vi "apply_settings.vi"(0 "Handle":i32, 1 "PreAmp Gain Control":string(combo), 3 "Trigger mode":string, 5 "ExposureTime":dbl=0.1, 7 "ElectronicShutteringMode":string(combo), 9 "AOI Height":i64, 11 "AOI Width":i64, 12 "Centre AOI":bool) -> (4 "AOIStride":i64, 6 "ImageSizeBytes":i64, 10 "Pixel Encoding":string, 14 "PixelData":u16[](array[numeric]), 15 "ByteData":u8[](array[numeric]))   [LabVIEW 2019]
panel:
  in  "Apply Settings":bool
  out "Ready":bool
  in  "Run":bool
  in  "error":errorcluster
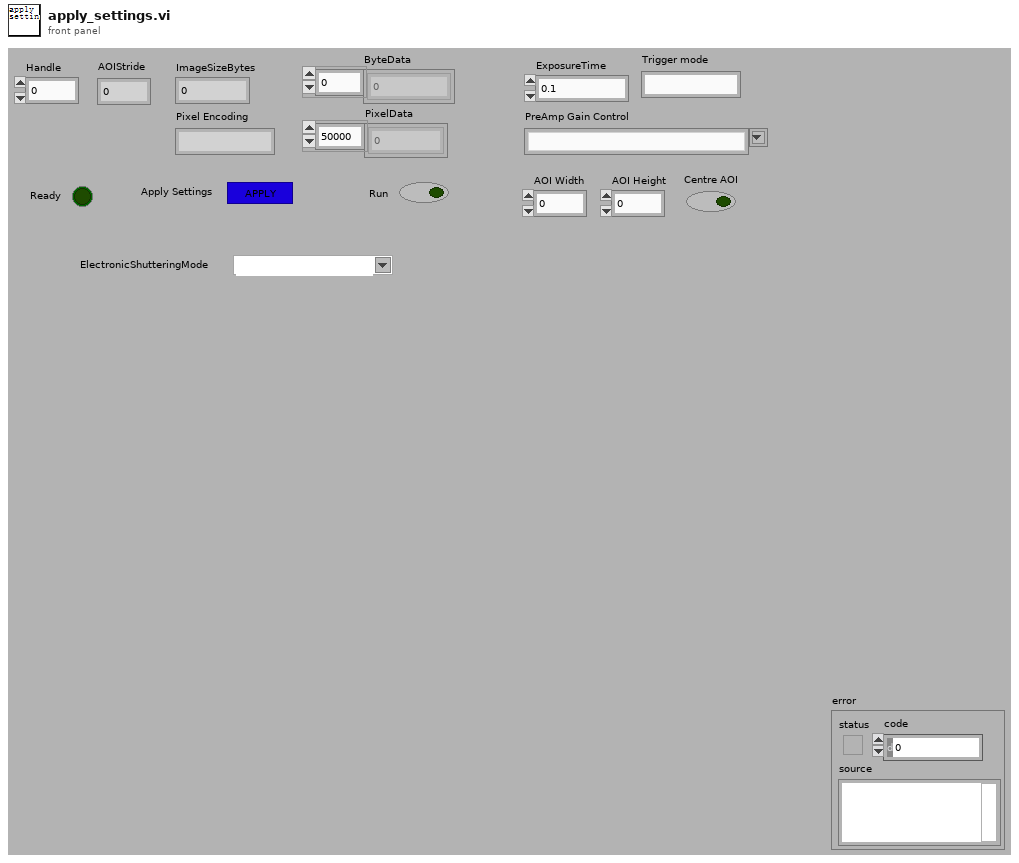
[diagram p1: front panel]
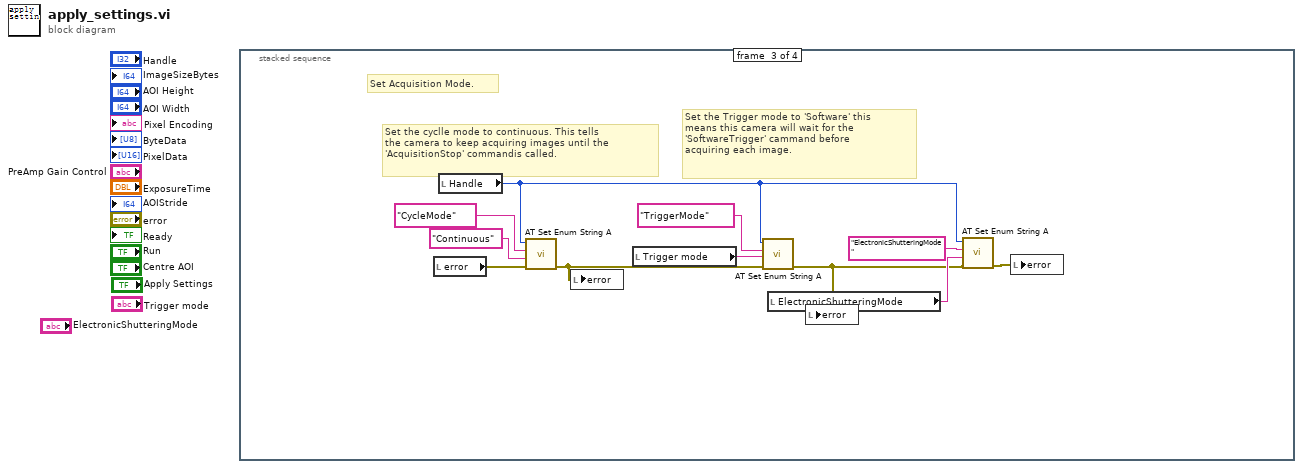
[diagram p0: block diagram]
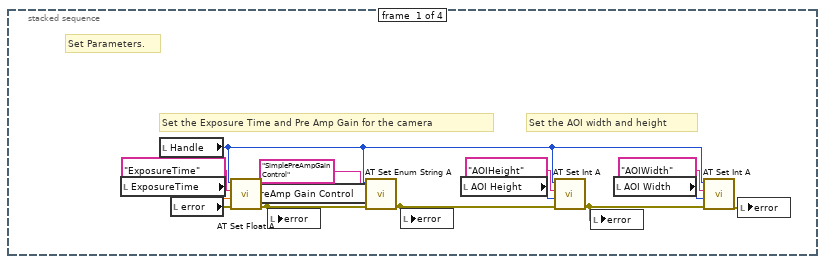
[diagram p2: hidden frame]
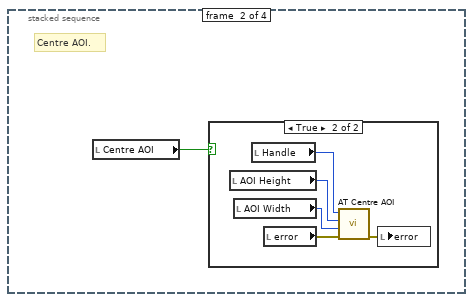
[diagram p3: hidden frame]
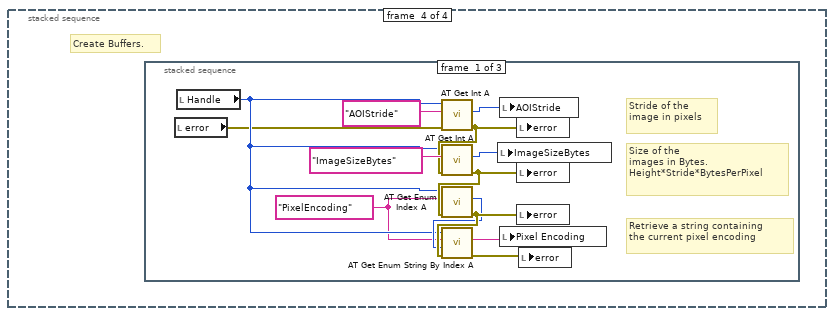
[diagram p5: hidden frame]
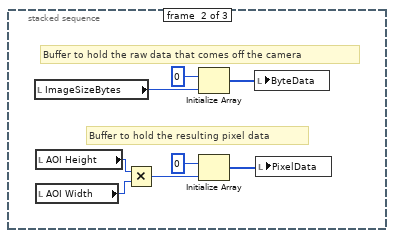
[diagram p6: hidden frame]
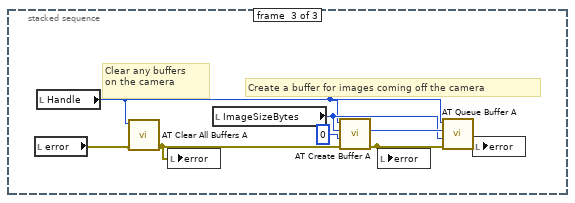
[diagram p7: hidden frame]
diagram:
  n1 = stacked-sequence {
    frame #0 {
      # "Set the AOI width and height"
      # "Set the Exposure Time and Pre Amp Gain for the camera"
      # "Set Parameters."
      n2 = local read "ExposureTime"() -> (w14:dbl)
      n3 = local read "Handle"() -> (w2:i32)
      n4 = local read "error"() -> (w10:errorcluster)
      n5 = call <userlib>:"AT Set Float A.vi"("error in (no error)"=w10, "Value"=w14, "Feature"="ExposureTime" ("ExposureTime"), "Hndl"=w2) -> ("error out"=w12:errorcluster)  [unwired: 6 in, 1 out]
      n6 = local read "PreAmp Gain Control"() -> (w13:string)
      n7 = local write "error"(w12) -> ()
      n8 = call <userlib>:"AT Set Enum String A.vi"("error in (no error)"=w12, "String"=w13, "Feature"="SimplePreAmpGainControl" ("Enum feature"), "Handle"=w2) -> ("error out"=w9:errorcluster)  [unwired: 6 in, 1 out]
      n9 = local write "error"(w9) -> ()
      n10 = local read "AOI Height"() -> (w6:i64)
      n11 = call <userlib>:"AT Set Int A.vi"("error in (no error)"=w9, "Value"=w6, "Feature"="AOIHeight" ("Integer feature"), "Handle"=w2) -> ("error out"=w7:errorcluster)  [unwired: 6 in, 1 out]
      n12 = local write "error"(w7) -> ()
      n13 = local read "AOI Width"() -> (w5:i64)
      n14 = call <userlib>:"AT Set Int A.vi"("error in (no error)"=w7, "Value"=w5, "Feature"="AOIWidth" ("Integer feature 2"), "Handle"=w2) -> ("error out"=w8:errorcluster)  [unwired: 6 in, 1 out]
      n15 = local write "error"(w8) -> ()
    }
    frame #1 {
      # "Centre AOI."
      n16 = local read "Centre AOI"() -> (w15:bool)
      n17 = case shown="True" w15 {
        frame False {
        }
        frame True {
          n18 = local read "AOI Height"() -> (w17:i64)
          n19 = local read "AOI Width"() -> (w18:i64)
          n20 = local read "Handle"() -> (w16:i32)
          n21 = local read "error"() -> (w19:errorcluster)
          n22 = call <userlib>:"AT Centre AOI.vi"("error in (no error)"=w19, "AOI Width"=w18, "AOI Height"=w17, "Handle"=w16) -> ("error out"=w20:errorcluster)  [unwired: 7 in]
          n23 = local write "error"(w20) -> ()
        }
      }
    }
    frame #2 {
      # "Set the Trigger mode to 'Software' this \nmeans this camera will wait for the \n'SoftwareTrigger' cammand before \nacquiring each image."
      # "Set the cyclle mode to continuous. This tells \nthe camera to keep acquiring images until the \n'AcquisitionStop' commandis called."
      # "Set Acquisition Mode."
      n24 = local read "error"() -> (w30:errorcluster)
      n25 = local read "Handle"() -> (w21:i32)
      n26 = call <userlib>:"AT Set Enum String A.vi"("error in (no error)"=w30, "String"="Continuous", "Feature"="CycleMode" ("Enum feature"), "Handle"=w21) -> ("error out"=w29:errorcluster)  [unwired: 6 in, 1 out]
      n27 = local write "error"(w29) -> ()
      n28 = local read "Trigger mode"() -> (w26:string)
      n29 = call <userlib>:"AT Set Enum String A.vi"("error in (no error)"=w29, "String"=w26, "Feature"="TriggerMode" ("Enum feature"), "Handle"=w21) -> ("error out"=w22:errorcluster)  [unwired: 6 in, 1 out]
      n30 = local read "ElectronicShutteringMode"() -> (w24:string)
      n31 = local write "error"(w22) -> ()
      n32 = call <userlib>:"AT Set Enum String A.vi"("error in (no error)"=w22, "String"=w24, "Feature"="ElectronicShutteringMode" ("Enum feature"), "Handle"=w21) -> ("error out"=w23:errorcluster)  [unwired: 6 in, 1 out]
      n33 = local write "error"(w23) -> ()
    }
    frame #3 {
      # "Create Buffers."
      n34 = stacked-sequence {
        frame #0 {
          w32 = "PixelEncoding" ("Enum feature")
          # "Retrieve a string containing \nthe current pixel encoding"
          # "Stride of the\nimage in pixels"
          # "Size of the\nimages in Bytes.\nHeight*Stride*BytesPerPixel"
          n35 = local read "error"() -> (w33:errorcluster)
          n36 = local read "Handle"() -> (w34:i32)
          n37 = call <userlib>:"AT Get Int A.vi"("error in (no error)"=w33, "Feature"="AOIStride" ("Integer feature"), "Handle"=w34) -> ("error out"=w40:errorcluster, "Value"=w44:i64)  [unwired: 6 in, 1 out]
          n38 = call <userlib>:"AT Get Int A.vi"("error in (no error)"=w40, "Feature"="ImageSizeBytes" ("Integer feature"), "Handle"=w34) -> ("error out"=w39:errorcluster, "Value"=w43:i64)  [unwired: 6 in, 1 out]
          n39 = call <userlib>:"AT Get Enum Index A.vi"("error in (no error)"=w39, "Feature"=w32, "Handle"=w34) -> ("error out"=w38:errorcluster, "Value"=w37:i32)  [unwired: 6 in, 1 out]
          n40 = call <userlib>:"AT Get Enum String By Index A.vi"("error in (no error)"=w38, "Index"=w37, "Feature"=w32, "Handle"=w34) -> ("error out"=w35:errorcluster, "String"=w36:string)  [unwired: 5 in, 1 out]
          n41 = local write "ImageSizeBytes"(w43) -> ()
          n42 = local write "AOIStride"(w44) -> ()
          n43 = local write "Pixel Encoding"(w36) -> ()
          n44 = local write "error"(w40) -> ()
          n45 = local write "error"(w39) -> ()
          n46 = local write "error"(w38) -> ()
          n47 = local write "error"(w35) -> ()
        }
        frame #1 {
          # "Buffer to hold the resulting pixel data"
          # "Buffer to hold the raw data that comes off the camera"
          n48 = local read "ImageSizeBytes"() -> (w46:i64)
          n49 = local read "AOI Height"() -> (w50:i64)
          n50 = local read "AOI Width"() -> (w51:i64)
          n51 = Multiply(x=w50, y=w51) -> (x*y=w45:i64)
          n52 = Initialize Array(u8 0, w46) -> (w48:u8[])
          n53 = Initialize Array(i64 0, w45) -> (w49:i64[])
          n54 = local write "ByteData"(w48) -> ()
          n55 = local write "PixelData"(w49) -> ()
        }
        frame #2 {
          # "Clear any buffers \non the camera"
          # "Create a buffer for images coming off the camera"
          n56 = local read "error"() -> (w55:errorcluster)
          n57 = local read "Handle"() -> (w53:i32)
          n58 = call <userlib>:"AT Clear All Buffers A.vi"("error in (no error)"=w55, "Handle"=w53) -> ("error out"=w54:errorcluster)  [unwired: 8 in, 1 out]
          n59 = local write "error"(w54) -> ()
          n60 = local read "ImageSizeBytes"() -> (w57:i64)
          n61 = call <userlib>:"AT Create Buffer A.vi"("error in (no error)"=w54, "Buffer"=0 ("Size"), "Size"=w57, "Handle"=w53) -> ("error out"=w59:errorcluster, "Buffer out"=w60:u64)  [unwired: 5 in, 1 out]
          n62 = local write "error"(w59) -> ()
          n63 = call <userlib>:"AT Queue Buffer A.vi"("error in (no error)"=w59, "PtrSize"=w57, "Ptr"=w60, "Handle"=w53) -> ("error out"=w56:errorcluster)  [unwired: 6 in, 1 out]
          n64 = local write "error"(w56) -> ()
        }
      }
    }
  }
